vi "flow-builder-io-write.vi"(6 "filenames.*":string[](array[string]), 7 "Step Name":string, 9 "Digital Timeout":u16, 10 "Value in":bool, 11 "Dout+AUX":string[](array[string])) -> (3 "Flow out":T2[](array[typedef]))   [LabVIEW 2024]
uses:
  controls/UiStepBuilder.ctl
  controls/type.step-builder.ctl
  controls/typeFlowBuilderDeviceGenerics.ctl
panel:
  in  "Device General Params":T1={"DoutTimeout"=2, "LoopInterval"=7}
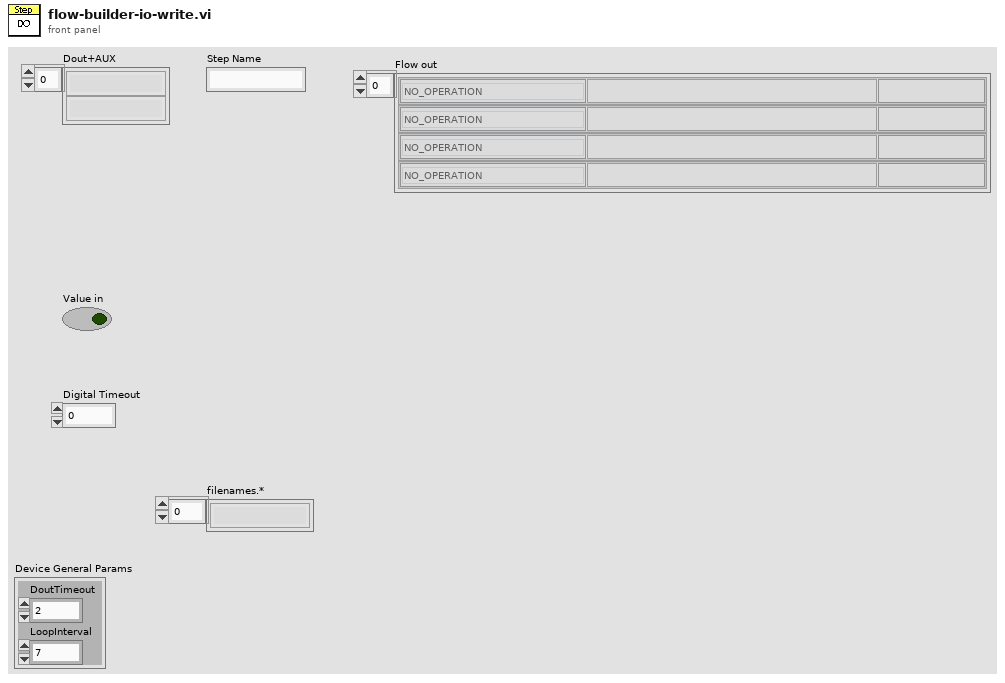
[diagram p1: front panel]
types:
  T1 = typedef "typeFlowBuilderDeviceGenerics.ctl" = cluster{"DoutTimeout":u16, "LoopInterval":u32}
  T2 = typedef "UiStepBuilder.ctl" = cluster{"Step Function":T3, "ParamString":string, "Step Label":string}
  T3 = typedef "type.step-builder.ctl" = enum16{"NO_OPERATION", "DELAY-JUMP", "DELAY", "JUMP", "COMPLETE", "SCHEDULER", "IRR-CHECK", "UNIT-CHECK", "UNIT-SAMPLE", "UNIT-DOSE", "LOG-REPORT", "LOG-MESSAGE", "IO-READ", "IO-READ-MANY", "IO-WRITE", "IO-COMPARE-OUT", "IO-COMPARE-IN", "PROC-START", "PROC-STOP", "PROC-LOAD", "PROC-IS-COMPLETED", "RECORD-MOVE", "GET-RH", "GET-UV", "GET-WD", "GET-WS", "OCS-CHECK", "OCS-RECORD"}
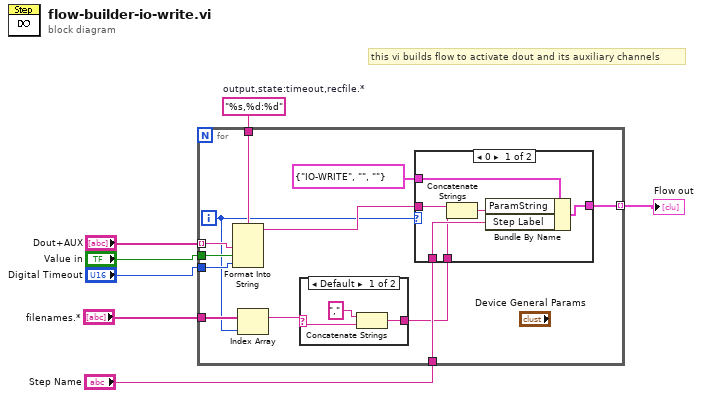
[diagram p0: block diagram]
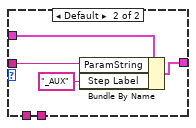
[diagram p3: hidden frame]
diagram:
  w2 = "%s,%d:%d"  # output,state:timeout,recfile.*
  # "this vi builds flow to activate dout and its auxiliary channels"
  n1 = for {
    tunnel: "Dout+AUX" -> [w17] mode=indexing
    tunnel: "Value in" -> [w16]
    tunnel: [w15] -> w6 mode=indexing
    tunnel: "Digital Timeout" -> [w14]
    tunnel: "Step Name" -> [w13]
    tunnel: w2 -> [w12]
    tunnel: "filenames.*" -> [w10]
    i -> [w8]
    n2 = Format Into String(format string=w12, w17, w16, w14) -> (resulting string=w18:string)  [unwired: 2 in, 1 out]
    n3 = Index Array(array=w10, index=w8) -> (element=w9:string)
    n4 = case shown="Default" w9 {
      selector: w9 -> [w22 _]
      tunnel: [w20 _] -> w11
      frame Default {
        n5 = Concatenate Strings("," ("string"), w22) -> (w20:string)
      }
      frame "" {
      }
    }
    n6 = case shown="0" w8 {
      tunnel: T2 {"Step Function"=enum."IO-WRITE", "ParamString"="", "Step Label"=""} ("FlowModeConstant 2") -> [w28 w32]
      tunnel: w18 -> [w27 w31]
      tunnel: [w26 w30] -> w15
      tunnel: w13 -> [w25 _]
      tunnel: w11 -> [w23 _]
      frame 0 {
        n7 = Concatenate Strings(w27, w23) -> (w24:string)
        n8 = Bundle By Name(cluster=w28, "ParamString"=w24, "Step Label"=w25) -> (w26:T2)
      }
      frame Default {
        n9 = Bundle By Name(cluster=w32, "ParamString"=w31, "Step Label"="_AUX") -> (w30:T2)
      }
    }
  }
  "Flow out" <- w6
